vi "题目6.7.vi"() -> ()   [LabVIEW 2017]
uses:
  <vilib>/Utility/file.llb/Read Delimited Spreadsheet (DBL).vi
  <vilib>/Analysis/NI_AALBase.lvlib
panel:
  out "波形图":dbl[](graph)
  out "all rows":dbl[][](array[numeric]) caption="所有行"
  out "拆分的路径":path
  in  "cycles":dbl=1.0 caption="周期" format="%0.2f"
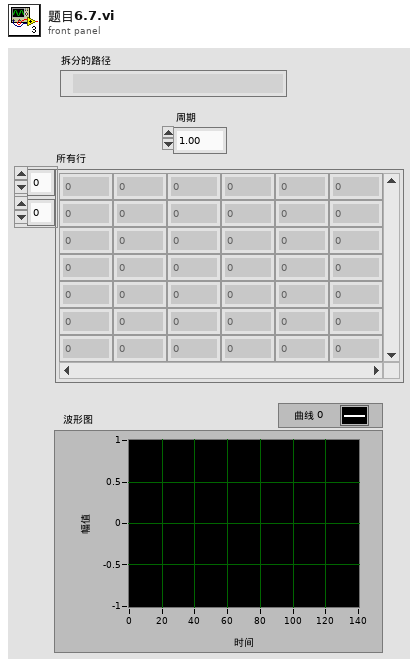
[diagram p1: front panel]
types:
  T1 = enum16{"open", "replace", "create", "open or create", "replace or create", "replace or create with confirmation"}
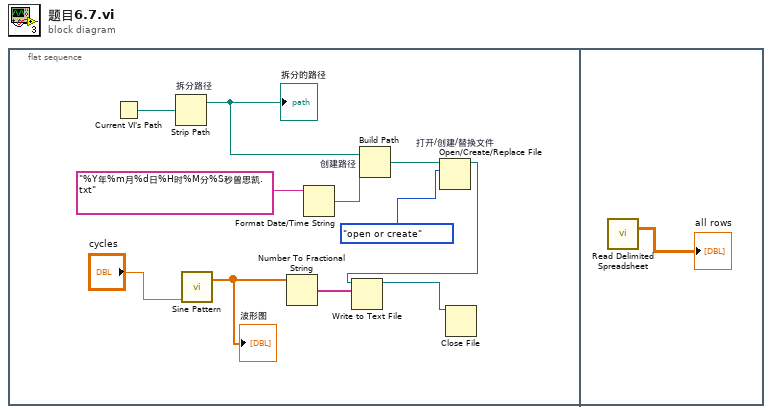
[diagram p0: block diagram]
diagram:
  n1 = flat-sequence {
    frame #0 {
      n2 = Current VI's Path() -> (path=w8:path)
      n3 = Strip Path "拆分路径"(path=w8) -> (stripped path=w9:path)  [unwired: 1 out]
      "拆分的路径" <- w9
      n4 = call <vilib>:"Sine Pattern.vi"("cycles"="cycles") -> ("Sinusoidal Pattern"=w4:dbl[])  [unwired: 3 in, 1 out]
      "波形图" <- w4
      n5 = Number To Fractional String(number=w4) -> (F-format string=w11:string[])  [unwired: 3 in]
      n6 = Format Date/Time String(time format string (%c)="%Y年%m月%d日%H时%M分%S秒曾思凯.txt" ("时间格式字符串(%c)")) -> (date/time string=w6:string)  [unwired: 2 in]
      n7 = Build Path "创建路径"(base path=w9, name or relative path=w6) -> (appended path=w5:path)
      n8 = Open/Create/Replace File "打开/创建/替换文件"(file path (use dialog)=w5, operation (0:open)=T1."open or create" ("操作(0:open)")) -> (refnum out=w2:refnum<file>)  [unwired: 4 in, 2 out]
      n9 = Write to Text File(file (use dialog)=w2, text=w11) -> (refnum out=w3:refnum<file>)  [unwired: 2 in, 2 out]
      n10 = Close File(refnum=w3) -> ()  [unwired: 1 in, 2 out]
    }
    frame #1 {
      n11 = call-poly <vilib>:"Read Delimited Spreadsheet.vi"() -> ("all rows"=→"all rows":dbl[][])  [unwired: 10 in, 5 out]
    }
  }
